vi "InitialConditionTest.vi"(0 "VI Reference In":refnum<vi>, 11 "error in":errorcluster) -> (4 "VI Reference Out":refnum<vi>, 15 "error out":errorcluster)   [LabVIEW 2016, in "Car Wash Test.lvlib"]
uses:
  Car Wash Test.lvlib
  Solution/Controls/Wash Options.ctl
  Solution/Controls/Car Wash Indicators.ctl
  main/apis/Assert/AssertControlDisable/AssertEnabled.vi
  main/apis/Assert/AssertControlValue/Equal.vi
  <vilib>/addons/_JKI Toolkits/Caraya/classes/Test/Test.lvclass
  main/Drona.lvlib
  main/apis/Assert/AssertControlValue/AssertControlValue.lvlib
  main/apis/Assert/AssertControlDisable/AssertControlDisable.lvlib
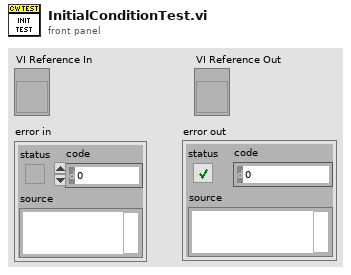
[diagram p1: front panel]
types:
  T1 = typedef "Car Wash Indicators.ctl" = cluster{"Under Body Wash":bool, "Bug Remover":bool, "Pre-Soak":bool, "High Pressure Wash":bool, "Low Pressure Wax":bool, "Spot Free Rinse":bool, "Tire Shine Foam":bool, "Air Dry":bool, "Vehicle Out of Position":bool}
  T2 = typedef "Wash Options.ctl" = cluster{"Under Body Wash":bool, "Bug Remover":bool, "Pre-Soak":bool, "High Pressure Wash":bool, "Low Pressure Wax":bool, "Spot Free Rinse":bool, "Tire Shine Foam":bool, "Air Dry":bool}
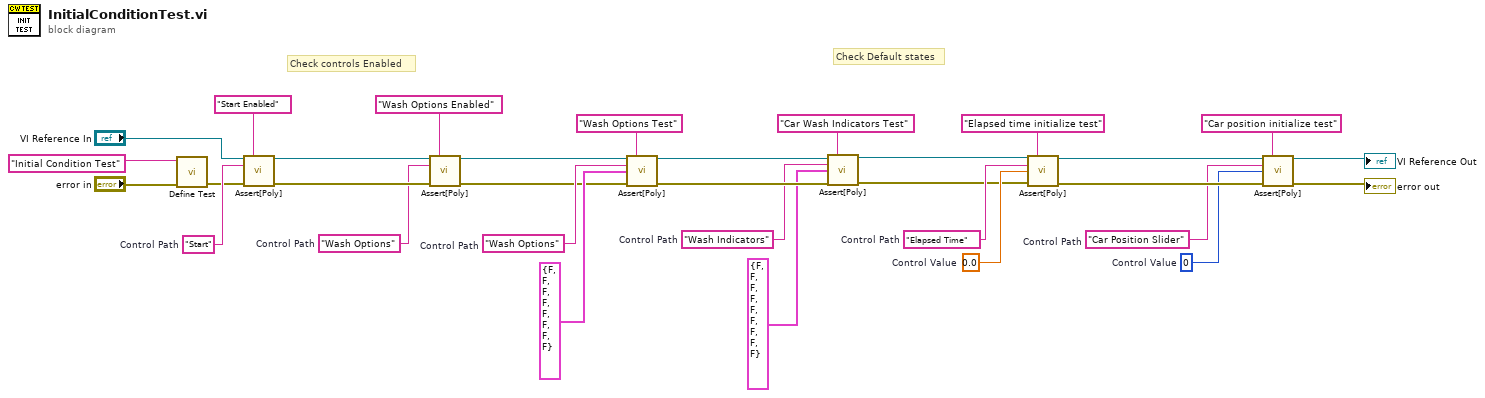
[diagram p0: block diagram]
diagram:
  w7 = "Start"  # Control Path
  w5 = "Wash Options"  # Control Path
  w17 = "Wash Indicators"  # Control Path
  w24 = "Wash Options"  # Control Path
  w25 = 0  # Control Value
  w26 = "Car Position Slider"  # Control Path
  w31 = 0.0  # Control Value
  w32 = "Elapsed Time"  # Control Path
  # "Check Default states"
  # "Check controls Enabled"
  n1 = call <vilib>:"Define Test.vi"("error in (no error)"="error in", "Label (VI Title)"="Initial Condition Test") -> ("error out"=w4:errorcluster)  [unwired: 9 in]
  n2 = call-poly "Assert[Poly].vi"("VI Reference In"="VI Reference In", "Label"="Start Enabled", "Control Path"=w7, "Error In"=w4) -> ("VI Reference Out"=w9:refnum<vi>, "Error Out"=w8:errorcluster)  [unwired: 10 in]
  n3 = call-poly "Assert[Poly].vi"("VI Reference In"=w9, "Label"="Wash Options Enabled", "Control Path"=w5, "Error In"=w8) -> ("VI Reference Out"=w1:refnum<vi>, "Error Out"=w3:errorcluster)  [unwired: 10 in]
  n4 = call-poly "Assert[Poly].vi"("VI Reference In"=w1, "Label"="Wash Options Test", "Control Path"=w24, "Control Value"=T2 {"Under Body Wash"=FALSE, "Bug Remover"=FALSE, "Pre-Soak"=FALSE, "High Pressure Wash"=FALSE, "Low Pressure Wax"=FALSE, "Spot Free Rinse"=FALSE, "Tire Shine Foam"=FALSE, "Air Dry"=FALSE} ("Wash Options"), "Error In"=w3) -> ("VI Reference Out"=w18:refnum<vi>, "Error Out"=w21:errorcluster)  [unwired: 9 in]
  n5 = call-poly "Assert[Poly].vi"("VI Reference In"=w18, "Label"="Car Wash Indicators Test", "Control Path"=w17, "Control Value"=T1 {"Under Body Wash"=FALSE, "Bug Remover"=FALSE, "Pre-Soak"=FALSE, "High Pressure Wash"=FALSE, "Low Pressure Wax"=FALSE, "Spot Free Rinse"=FALSE, "Tire Shine Foam"=FALSE, "Air Dry"=FALSE, "Vehicle Out of Position"=FALSE} ("Car Wash Indicators"), "Error In"=w21) -> ("VI Reference Out"=w19:refnum<vi>, "Error Out"=w20:errorcluster)  [unwired: 9 in]
  n6 = call-poly "Assert[Poly].vi"("VI Reference In"=w19, "Label"="Elapsed time initialize test", "Control Path"=w32, "Control Value"=w31, "Error In"=w20) -> ("VI Reference Out"=w27:refnum<vi>, "Error Out"=w28:errorcluster)  [unwired: 9 in]
  n7 = call-poly "Assert[Poly].vi"("VI Reference In"=w27, "Label"="Car position initialize test", "Control Path"=w26, "Control Value"=w25, "Error In"=w28) -> ("VI Reference Out"=→"VI Reference Out":refnum<vi>, "Error Out"=→"error out":errorcluster)  [unwired: 9 in]
